vi "React Polymer.vi"(8 "Error In":errorcluster, 10 "Redux Element":string, 11 "Unreacted Polymer":string) -> (0 "Error Out":errorcluster, 2 "Size of Polymer":i32, 3 "Polymer":string)   [LabVIEW 2019]
doc: "Remove all instances of adjacent characters where their cases differ (e.g. aA bB Cc) but not where they're the same (e.g. AA bb CC).\n\nIf a redux element is provided, this VI will remove all instances of that character prior to performing the reaction."
uses:
  <vilib>/Utility/error.llb/Error Cluster From Error Code.vi
  <vilib>/ErrorRing/Error Ring.xnode
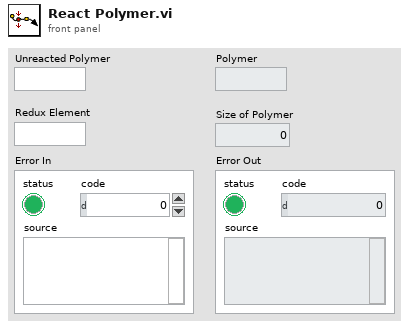
[diagram p1: front panel]
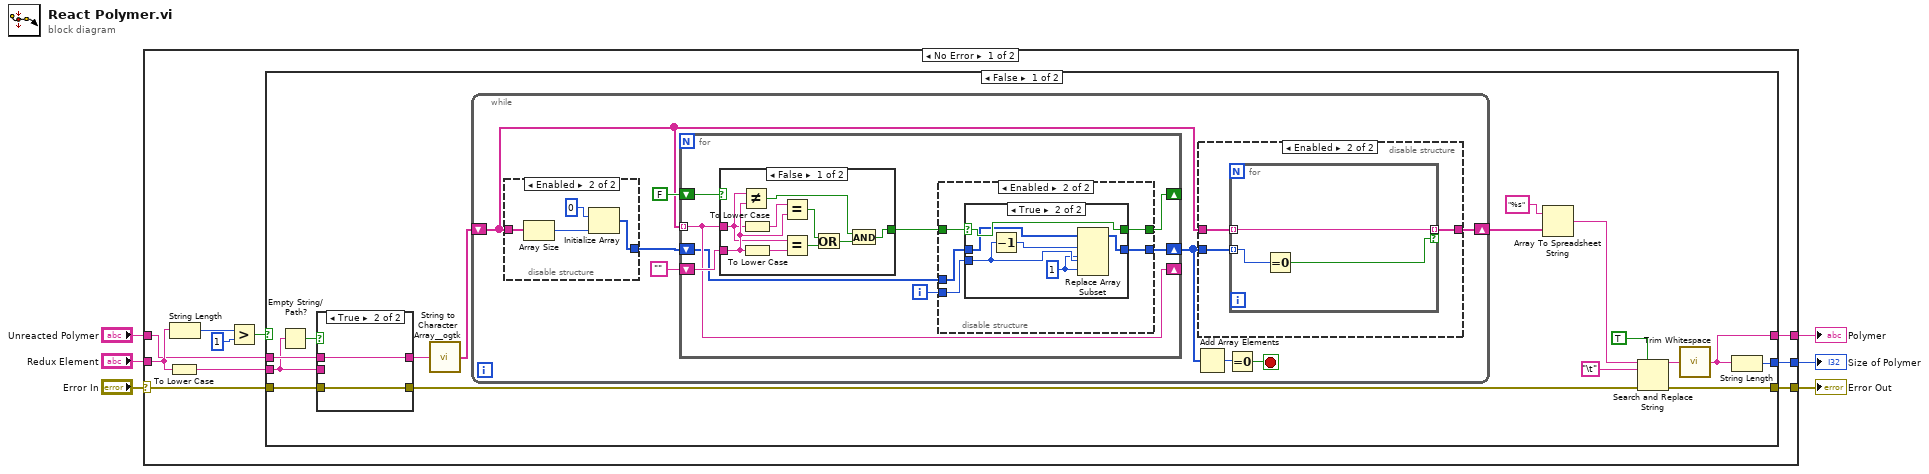
[diagram p0: block diagram]
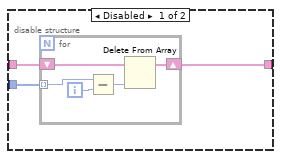
[diagram p2: hidden frame]
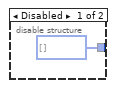
[diagram p3: hidden frame]
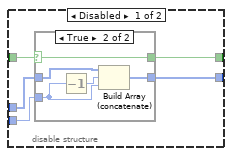
[diagram p4: hidden frame]
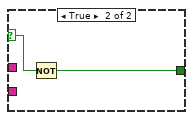
[diagram p7: hidden frame]
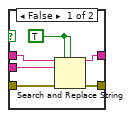
[diagram p8: hidden frame]
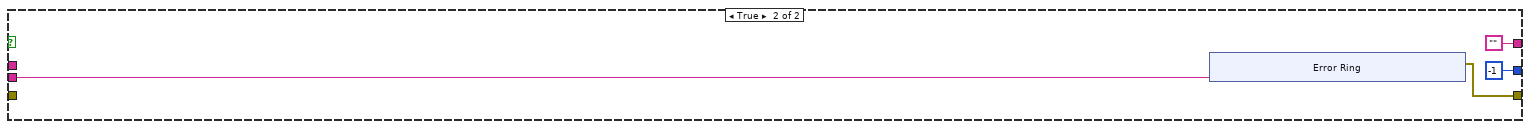
[diagram p9: hidden frame]
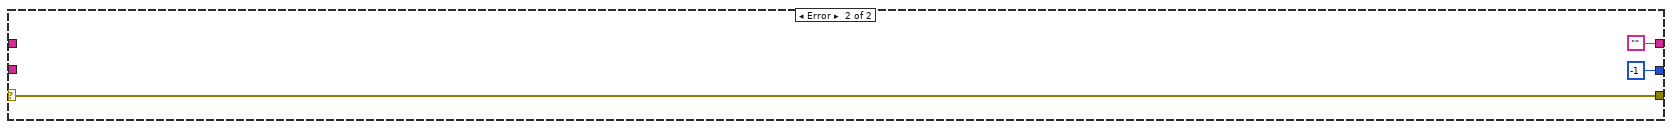
[diagram p10: hidden frame]
diagram:
  n1 = case shown="No Error" "Error In" {
    selector: "Error In" -> [w14 w123]
    tunnel: [w16 ""] -> w6
    tunnel: [w15 -1] -> w5
    tunnel: "Unreacted Polymer" -> [w7 _]
    tunnel: [w13 w123] -> w2
    tunnel: "Redux Element" -> [w11 _]
    frame No Error {
      n2 = To Lower Case(string=w11) -> (all lower case string=w12:string)
      n3 = String Length(string=w11) -> (length=w10:i32)
      n4 = Greater?(x=w10, y=1) -> (0:w8:bool)
      n5 = case shown="False" w8 {
        tunnel: [w32 ""] -> w16
        tunnel: [w30 -1] -> w15
        tunnel: w14 -> [w18 _]
        tunnel: [w24 w115] -> w13
        tunnel: w12 -> [w20 w112]
        tunnel: w7 -> [w23 _]
        frame False {
          n6 = Empty String/Path?(string/path=w20) -> (empty?=w21:bool)
          n7 = case shown="True" w21 {
            tunnel: w20 -> [w109 _]
            tunnel: w23 -> [w108 w111]
            tunnel: [w107 w111] -> w19
            tunnel: w18 -> [w106 w110]
            tunnel: [w105 w110] -> w17
            frame False {
              w104 = TRUE ("replace all? (F)")
              n8 = Search and Replace String(replace all?=w104, case sensitive?=w104, input string=w108, search string=w109, error in=w106) -> (result string=w107:string, error out=w105:errorcluster)  [unwired: 3 in, 2 out]
            }
            frame True {
            }
          }
          n9 = call <userlib>:"String to Character Array__ogtk.vi"("Input String"=w19) -> ("Character Array"=w22:string[])
          n10 = while {
            shift-right: [w37] -> w25
            shift-left: w22 -> [w36]
            stop <- w33 stop-if-true
            n11 = disable-structure shown="Enabled" {
              disable-tunnel: [i32[] [] w56] -> w38
              disable-tunnel: w36 -> [_ w59]
              frame Disabled {
              }
              frame Enabled {
                n12 = Array Size(array=w59) -> (size(s)=w58:i32)
                n13 = Initialize Array(0 ("element"), w58) -> (w56:i32[])
              }
            }
            n14 = for {
              tunnel: w36 -> [w66] mode=indexing
              shift-right: [w66] -> _
              shift-left: "" -> [w67]
              shift-right: [w63] -> _
              shift-left: FALSE -> [w65]
              shift-right: [w60] -> w35
              shift-left: w38 -> [w62]
              i -> [w61]
              n15 = case shown="False" w65 {
                selector: w65 -> [_ w103]
                tunnel: w67 -> [w101 _]
                tunnel: w66 -> [w97 _]
                tunnel: [w93 w102] -> w64
                frame False {
                  n16 = Not Equal?(x=w97, y=w101) -> (x != y?=w95:bool)
                  n17 = To Lower Case(string=w97) -> (all lower case string=w96:string)
                  n18 = To Lower Case(string=w101) -> (all lower case string=w98:string)
                  n19 = Equal?(x=w96, y=w101) -> (x = y?=w99:bool)
                  n20 = Equal?(x=w97, y=w98) -> (x = y?=w100:bool)
                  n21 = Or(x=w99, y=w100) -> (x .or. y?=w94:bool)
                  n22 = And(x=w95, y=w94) -> (x .and. y?=w93:bool)
                }
                frame True {
                  n23 = Not(x=w103) -> (.not. x?=w102:bool)
                }
              }
              n24 = disable-structure shown="Enabled" {
                disable-tunnel: w64 -> [w72 w82]
                disable-tunnel: [w71 w81] -> w63
                disable-tunnel: w62 -> [w70 w84]
                disable-tunnel: w61 -> [w69 w83]
                disable-tunnel: [w68 w80] -> w60
                frame Disabled {
                  n25 = case shown="True" w72 {
                    selector: w72 -> [w74 w79]
                    tunnel: [w74 w79] -> w71
                    tunnel: w70 -> [w73 w78]
                    tunnel: w69 -> [_ w75]
                    tunnel: [w73 w77] -> w68
                    frame False {
                    }
                    frame True {
                      n26 = Decrement(x=w75) -> (x-1=w76:i32)
                      n27 = Build Array (concatenate)(w78, w76, w75) -> (w77:i32[])
                    }
                  }
                }
                frame Enabled {
                  n28 = case shown="True" w82 {
                    selector: w82 -> [w86 w92]
                    tunnel: [w86 w92] -> w81
                    tunnel: w84 -> [w85 w91]
                    tunnel: w83 -> [_ w90]
                    tunnel: [w85 w87] -> w80
                    frame False {
                    }
                    frame True {
                      w88 = 1 ("new element/subarray")
                      n29 = Decrement(x=w90) -> (x-1=w89:i32)
                      n30 = Replace Array Subset(array=w91, new element #1=w88, index #1=w89, new element #2=w88, index #2=w90) -> (w87:i32[])
                    }
                  }
                }
              }
            }
            n31 = Add Array Elements(numeric array=w35) -> (sum=w34:i32)
            n32 = disable-structure shown="Enabled" {
              disable-tunnel: w35 -> [w43 w50]
              disable-tunnel: [w42 w49] -> w37
              disable-tunnel: w36 -> [w41 w51]
              frame Disabled {
                n33 = for {
                  tunnel: w43 -> [w48] mode=indexing
                  shift-right: [w45] -> w42
                  shift-left: w41 -> [w46]
                  i -> [w47]
                  n34 = Subtract(x=w48, y=w47) -> (x-y=w44:i32)
                  n35 = Delete From Array(array=w46, index=w44) -> (array with subset deleted=w45:string[])  [unwired: 1 in, 1 out]
                }
              }
              frame Enabled {
                n36 = for {
                  tunnel: w50 -> [w54] mode=indexing
                  tunnel: w51 -> [w53] mode=indexing
                  tunnel: [w53] -> w49 mode=indexing if=w52
                  n37 = Equal To 0?(x=w54) -> (x = 0?=w52:bool)
                }
              }
            }
            n38 = Equal To 0?(x=w34) -> (x = 0?=w33:bool)
          }
          n39 = Array To Spreadsheet String(array=w25, 3:"%s" ("format string")) -> (spreadsheet string=w28:string)  [unwired: 1 in]
          n40 = Search and Replace String(replace all?=TRUE ("replace all? (F)"), input string=w28, search string="\t", error in=w17) -> (result string=w31:string, error out=w24:errorcluster)  [unwired: 4 in, 2 out]
          n41 = call <vilib>:"Trim Whitespace.vi"("string"=w31) -> ("trimmed string"=w32:string)  [unwired: 1 in]
          n42 = String Length(string=w32) -> (length=w30:i32)
        }
        frame True {
          n43 = xnode "Error Ring"("parameter 0"=w112) -> ("error out"=w115:errorcluster)
        }
      }
    }
    frame Error {
    }
  }
  "Polymer" <- w6
  "Size of Polymer" <- w5
  "Error Out" <- w2
